vi "Create Observer (array).vi"(8 "Additional Input":refnum<class "Send.lvclass">, 9 "Array of Input":refnum<class "Send.lvclass">[](array[class])) -> (3 "Observer":refnum<class "Observer.lvclass">)   [LabVIEW 2011, in "Messenging.lvlib" / "ObserverSet.lvclass"]
uses:
  ObserverSet.lvclass
  SendOnly/Observer.lvclass
  Send/Send.lvclass
  ObserverSet.lvclass/ObserverSet.ctl
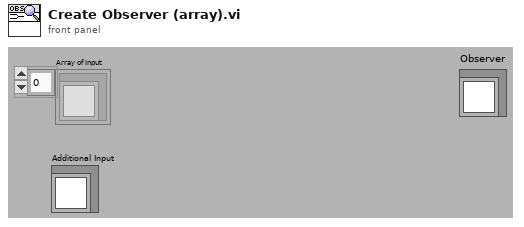
[diagram p1: front panel]
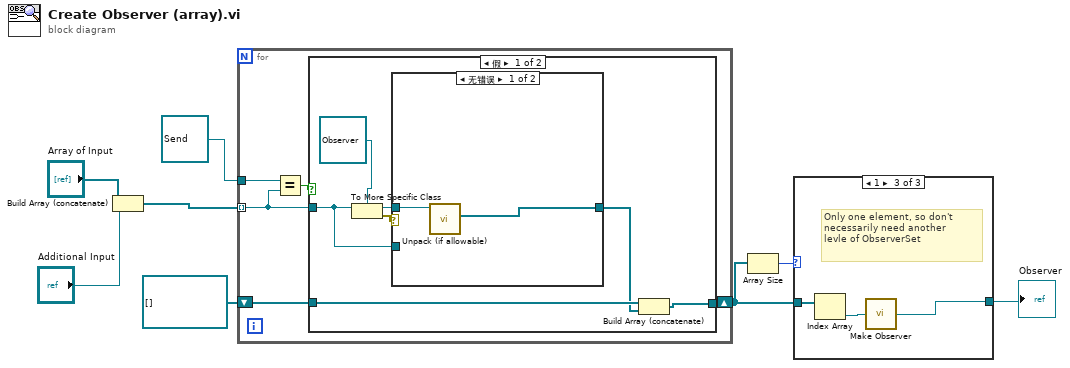
[diagram p0: block diagram]
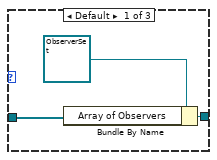
[diagram p2: hidden frame]
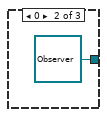
[diagram p3: hidden frame]
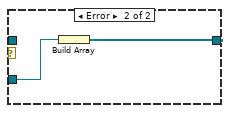
[diagram p4: hidden frame]
diagram:
  n1 = Build Array (concatenate)("Array of Input", "Additional Input") -> (w6:refnum<class "Send.lvclass">[])
  n2 = for {
    tunnel: w6 -> [w12] mode=indexing
    shift-right: [w9] -> w1
    shift-left: refnum<class "Send.lvclass">[] [] -> [w13]
    tunnel: refnum<class "Send.lvclass"> refnum ("Messenging.lvlib:Send.lvclass") -> [w11]
    n3 = Equal?(x=w11, y=w12) -> (x = y?=w10:bool)
    n4 = case shown="假" w10 {
      tunnel: [w20 w25] -> w9
      tunnel: w13 -> [w19 w25]
      tunnel: w12 -> [w14 _]
      frame False {
        n5 = To More Specific Class(target class=refnum<class "Observer.lvclass"> refnum ("Messenging.lvlib:Observer.lvclass"), reference=w14) -> (specific class reference=w17:refnum<class "Observer.lvclass">, error out=w18:errorcluster)  [unwired: 1 in]
        n6 = case shown="无错误" w18 {
          tunnel: w17 -> [w22 _]
          tunnel: [w21 w24] -> w16
          tunnel: w14 -> [_ w23]
          frame No Error {
            n7 = call-dynamic "Unpack (if allowable).vi"("Observer in"=w22) -> ("Array out"=w21:refnum<class "Send.lvclass">[])  [unwired: 10 out]
          }
          frame Error {
            n8 = Build Array(w23) -> (w24:refnum<class "Send.lvclass">[])
          }
        }
        n9 = Build Array (concatenate)(w19, w16) -> (w20:refnum<class "Send.lvclass">[])
      }
      frame True {
        # "Drop Null Messengers (unconnected inputs)"
      }
    }
  }
  n10 = Array Size(array=w1) -> (size(s)=w2:i32)
  n11 = case shown="1" w2 {
    tunnel: w1 -> [w28 _ w32]
    tunnel: [w27 refnum<class "Observer.lvclass"> refnum ("Observer") w30] -> w3
    frame Default {
      n12 = Bundle By Name(cluster=refnum<class "ObserverSet.lvclass"> refnum ("SendMultiple in"), "Array of Observers"=w28) -> (w27:refnum<class "ObserverSet.lvclass">)
    }
    frame 0 {
    }
    frame 1 {
      # "Only one element, so don't\nnecessarily need another\nlevle of ObserverSet"
      n13 = Index Array(array=w32) -> (element=w31:refnum<class "Send.lvclass">)  [unwired: 1 in]
      n14 = call "Make Observer.vi"("To be an Observer"=w31) -> ("Observer"=w30:refnum<class "Observer.lvclass">)
    }
  }
  "Observer" <- w3
